vi "33120SyncStat.vi"(4 "error in (no error)":errorcluster, 6 "Turn off Sync?":bool, 7 "VISA session in":refnum<visa-resource-name>) -> (0 "error out":errorcluster, 3 "VISA session out":refnum<visa-resource-name>)   [LabVIEW 2022 SP3]
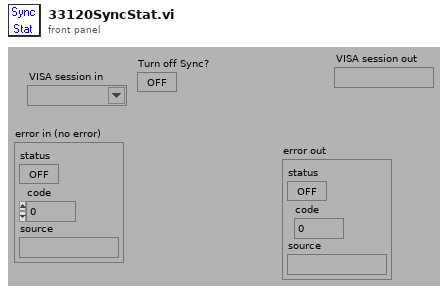
[diagram p1: front panel]
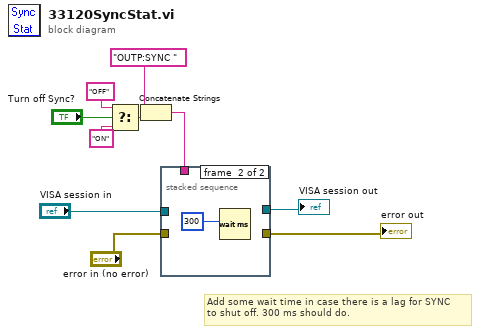
[diagram p0: block diagram]
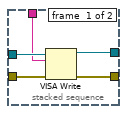
[diagram p2: hidden frame]
diagram:
  # "Add some wait time in case there is a lag for SYNC\nto shut off. 300 ms should do."
  n1 = Select(t="OFF", s="Turn off Sync?", f="ON") -> (s? t:f=w5:string)
  n2 = Concatenate Strings("OUTP:SYNC ", w5) -> (w4:string)
  n3 = stacked-sequence {
    tunnel: "VISA session in" -> [w15 _]
    tunnel: [w14 _] -> w10
    tunnel: [w13 _] -> w2
    tunnel: w4 -> [w12 _]
    tunnel: "error in (no error)" -> [w11 _]
    frame #0 {
      n4 = VISA Write(VISA resource name=w15, write buffer=w12, error in (no error)=w11) -> (VISA resource name out=w14:refnum<visa-resource-name>, error out=w13:errorcluster)  [unwired: 1 out]
    }
    frame #1 {
      n5 = Wait (ms)(milliseconds to wait=300) -> ()  [unwired: 1 out]
    }
  }
  "error out" <- w2
  "VISA session out" <- w10
